vi "DataTranslation_Differential.vi"() -> ()   [LabVIEW 2011]
uses:
  Globals/Meas_global.vi
  PWA/PWAtasksGLOBAL.vi
  Data_Translation/DataTranslation_global.vi
  <userlib>/LV-Link3/PolySubVIs/DtOLTimingSetInput.vi
  <userlib>/LV-Link3/PolySubVIs/DtCreateAinChan.vi
  <userlib>/LV-Link3/PolySubVIs/DtOLReadMultiple2D.vi
  <userlib>/LV-Link3/PolySubVIs/DtOLTriggerDigital.vi
panel:
  out "Waveform Graph":dbl[][](graph)
  out "error out":errorcluster={"status"=TRUE, "code"=1172, "source"="Error calling method LvLink2.LvTask.ReadDblData2DAs1D, (System.Reflection.TargetInvocationException: Exception has been thrown by the target of an invocation.\n\tInner Exception: LvLink2.LvException: Timeout) <append><b>LvLink2.LvException</b> in OLReadMultiple2D.vi->DataTranslation_server.vi->Acquire_Data.vi->Get_data.vi->Measurement.vi"}
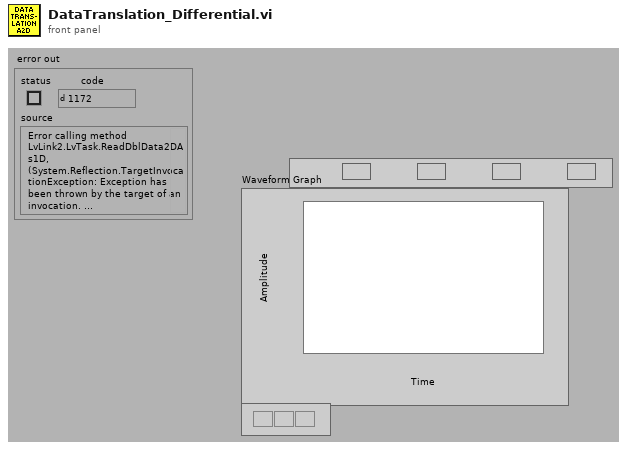
[diagram p1: front panel]
types:
  T1 = typedef "Ch_and_Spans.ctl" = cluster{"high limit (10V)":sgl, "low limit (-10V)":sgl, "Ch No":i16, "Var name":string, "Use Latest Calib":bool}
  T2 = typedef "Trigger_Mode.ctl" = enum16{"Free Running", "Start on Trigger", "Trigger Every Block", "Trigger Every Sample"}
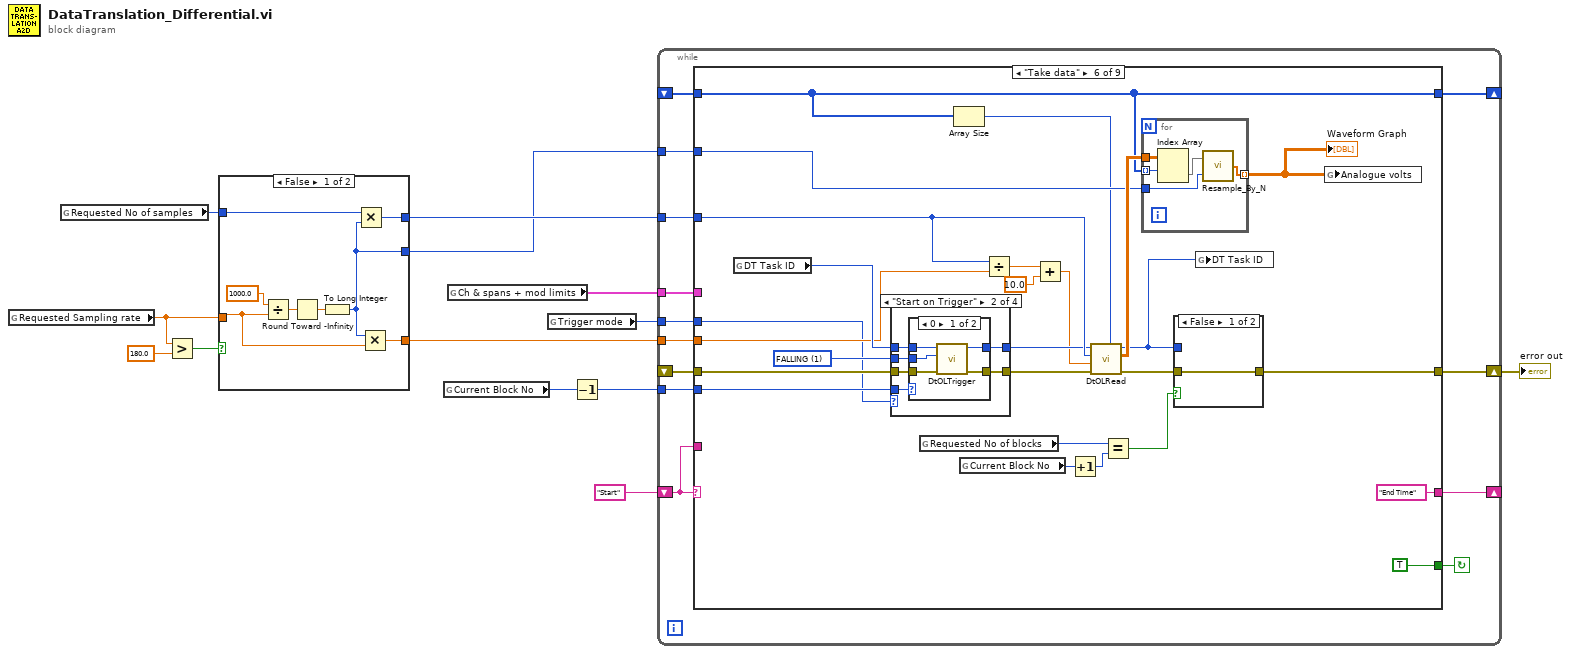
[diagram p0: block diagram]
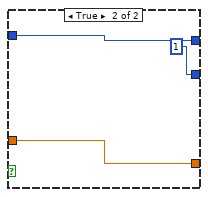
[diagram p2: hidden frame]
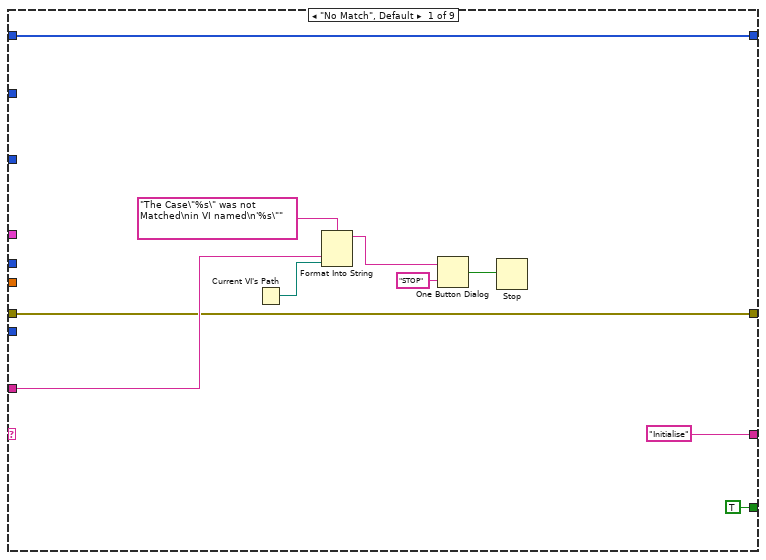
[diagram p3: hidden frame]
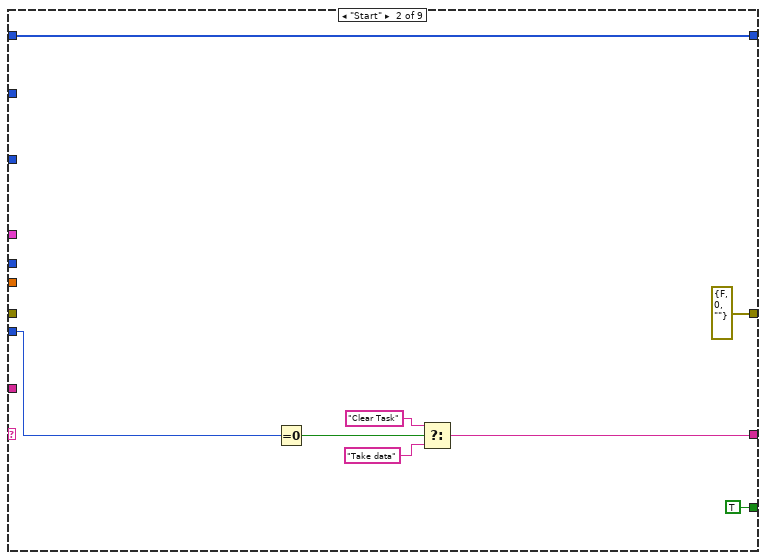
[diagram p4: hidden frame]
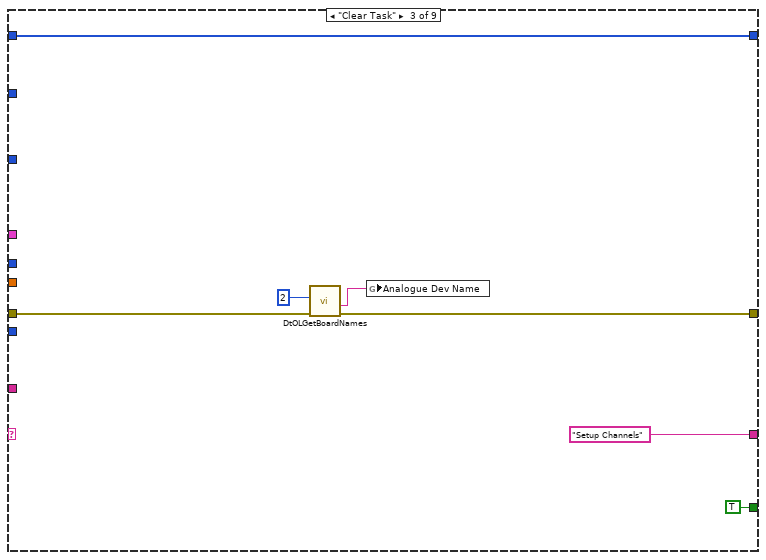
[diagram p5: hidden frame]
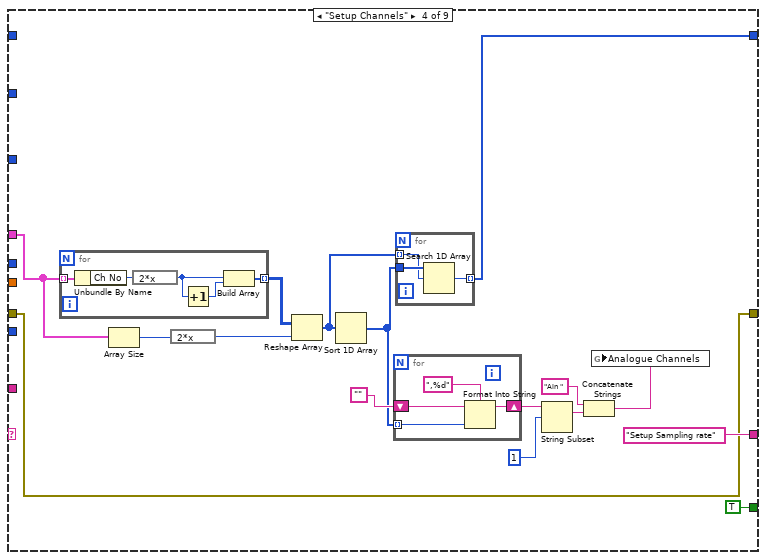
[diagram p6: hidden frame]
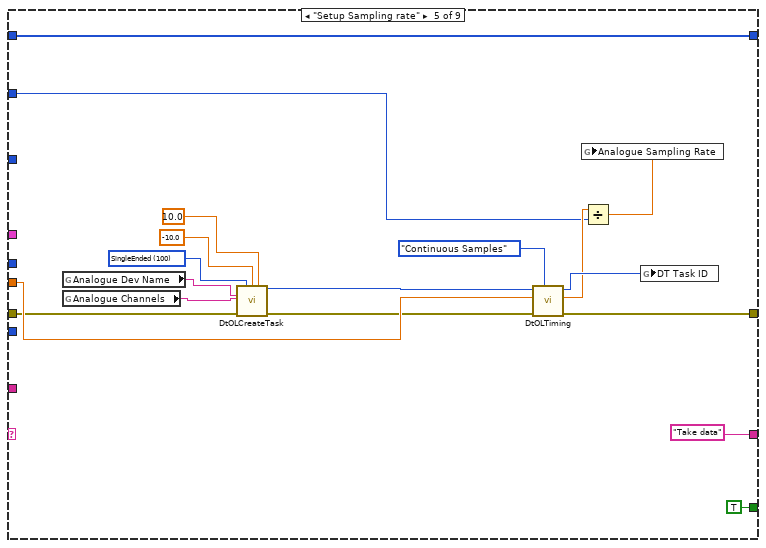
[diagram p7: hidden frame]
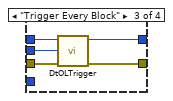
[diagram p10: hidden frame]
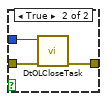
[diagram p12: hidden frame]
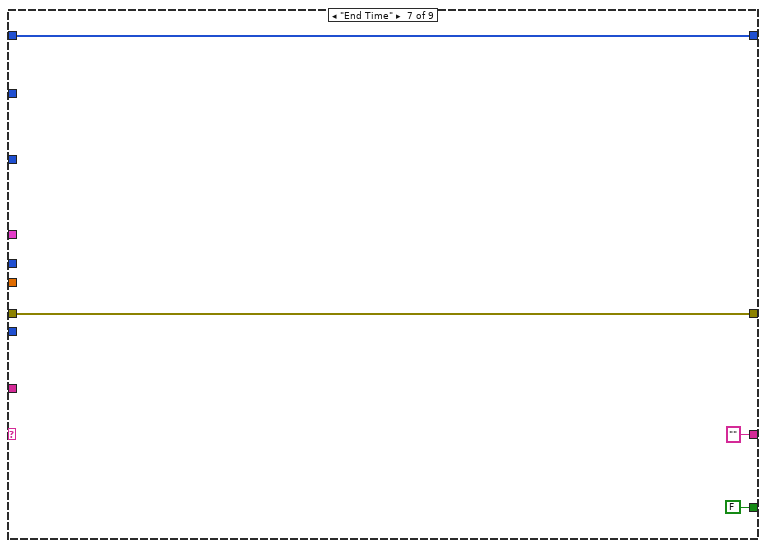
[diagram p13: hidden frame]
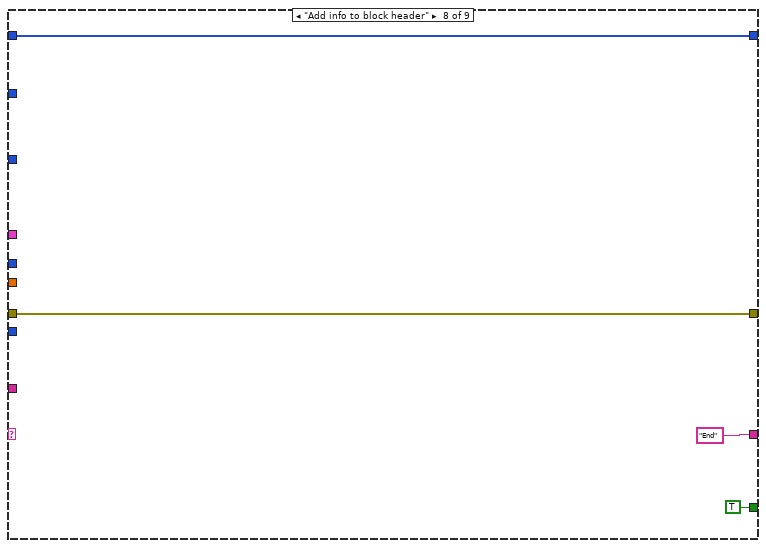
[diagram p14: hidden frame]
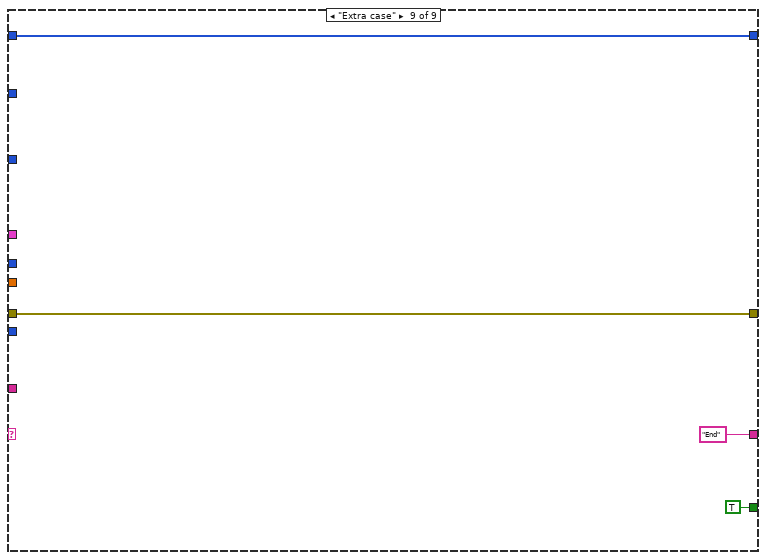
[diagram p15: hidden frame]
diagram:
  n1 = global read "Meas_global.vi" "Requested Sampling rate"() -> (w5:dbl)
  n2 = global read "Meas_global.vi" "Requested No of samples"() -> (w2:i32)
  n3 = Greater?(x=w5, y=180.0) -> (0:w10:bool)
  n4 = case shown="False" w10 {
    tunnel: w5 -> [w15 w24]
    tunnel: [w16 w24] -> w9
    tunnel: [w18 w23] -> w8
    tunnel: w2 -> [w17 w23]
    tunnel: [w14 1] -> w7
    frame False {
      n5 = Divide(x=1000.0, y=w15) -> (x/y=w20:dbl)
      n6 = Round Toward -Infinity(1:w20) -> (0:w19:dbl)
      n7 = To Long Integer(number=w19) -> (32bit integer=w14:i32)
      n8 = Multiply(x=w17, y=w14) -> (x*y=w18:i32)
      n9 = Multiply(x=w14, y=w15) -> (x*y=w16:dbl)
    }
    frame True {
    }
  }
  n10 = global read "Meas_global.vi" "Current Block No"() -> (w4:i32)
  n11 = global read "Meas_global.vi" "Ch & spans + mod limits"() -> (w6:T1[])
  n12 = global read "Meas_global.vi" "Trigger mode"() -> (w1:T2)
  n13 = Decrement(x=w4) -> (x-1=w3:i32)
  n14 = while {
    shift-left: "Start" -> [w36]
    shift-right: [w37] -> _
    shift-right: [w30] -> w12
    shift-left: _ -> [w35]
    tunnel: w9 -> [w34]
    tunnel: w8 -> [w33]
    tunnel: w3 -> [w32]
    tunnel: w6 -> [w31]
    shift-right: [w29] -> _
    shift-left: _ -> [w28]
    tunnel: w7 -> [w27]
    tunnel: w1 -> [w25]
    stop <- w26 continue-if-true
    n15 = case shown="\"Take data\"" w36 {
      tunnel: ["Initialise" w53 "Setup Channels" "Setup Sampling rate" "Take data" "End Time" "" ("f") "End" ("f") "End" ("f")] -> w37
      tunnel: w36 -> [w43 _ _ _ _ _ _ _ _]
      tunnel: [w40 errorcluster {"status"=FALSE, "code"=0, "source"=""} ("error out") w57 w72 w108 w119 w169 w172 w176] -> w30
      tunnel: w35 -> [w40 _ w58 w72 w94 w133 w169 w172 w176]
      tunnel: w34 -> [_ _ _ _ w107 w129 _ _ _]
      tunnel: w33 -> [_ _ _ _ _ w130 _ _ _]
      tunnel: w32 -> [_ w55 _ _ _ w128 _ _ _]
      tunnel: w31 -> [_ _ _ w66 _ _ _ _ _]
      tunnel: [w39 w51 w61 w74 w105 w127 w168 w171 w175] -> w29
      tunnel: w28 -> [w39 w51 w61 _ w105 w127 w168 w171 w175]
      tunnel: w27 -> [_ _ _ _ w102 w126 _ _ _]
      tunnel: [TRUE TRUE TRUE TRUE TRUE TRUE FALSE TRUE TRUE] -> w26
      tunnel: w25 -> [_ _ _ _ _ w111 _ _ _]
      frame "No Match", Default {
        (unwired) FALSE
        n16 = Current VI's Path() -> (path=w42:path)
        n17 = Format Into String(format string="The Case\"%s\" was not Matched\nin VI named\n'%s\"" ("Format String"), w43, w42) -> (resulting string=w46:string)  [unwired: 2 in, 1 out]
        n18 = One Button Dialog(message=w46, button name ("OK")="STOP") -> (true=w44:bool)
        n19 = Stop(stop? (T)=w44) -> ()
      }
      frame "Start" {
        (unwired) TRUE
        n20 = Equal To 0?(x=w55) -> (x = 0?=w54:bool)
        n21 = Select(t="Clear Task", s=w54, f="Take data") -> (s? t:f=w53:string)
      }
      frame "Clear Task" {
        (unwired) TRUE
        n22 = call <userlib>:"DtOLGetBoardNames.vi"("error in (no error)"=w58, "Select Board"=u32 2) -> ("error out"=w57:errorcluster, "Board Name"=w59:string)  [unwired: 7 in, 1 out]
        n23 = global write "PWAtasksGLOBAL.vi" "Analogue Dev Name"(w59) -> ()
      }
      frame "Setup Channels" {
        (unwired) TRUE
        n24 = for {
          tunnel: [w89] -> w69 mode=indexing
          tunnel: w66 -> [w88] mode=indexing
          n25 = Unbundle By Name(w88) -> ("Ch No"=w87:i16)
          n26 = expression code="2*x"(w87) -> (w86:i16)
          n27 = Increment(x=w86) -> (x+1=w90:i16)
          n28 = Build Array(w86, w90) -> (w89:i16[])
        }
        n29 = Array Size(array=w66) -> (size(s)=w68:i32)
        n30 = expression code="2*x"(w68) -> (w67:i32)
        n31 = Reshape Array(w69, w67) -> (w65:i16[])
        n32 = Sort 1D Array(array=w65) -> (sorted array=w63:i16[])
        n33 = for {
          shift-right: [w80] -> w64
          shift-left: "" -> [w81]
          tunnel: w63 -> [w79] mode=indexing
          n34 = Format Into String(format string=",%d", initial string=w81, w79) -> (resulting string=w80:string)  [unwired: 1 in, 1 out]
        }
        n35 = for {
          tunnel: w63 -> [w85]
          tunnel: w65 -> [w84] mode=indexing
          tunnel: [w83] -> w74 mode=indexing
          n36 = Search 1D Array(1D array=w85, element=w84) -> (index of element=w83:i32)  [unwired: 1 in]
        }
        n37 = String Subset(string=w64, offset (0)=1) -> (substring=w76:string)  [unwired: 1 in]
        n38 = Concatenate Strings("Ain ", w76) -> (w71:string)
        n39 = global write "Meas_global.vi" "Analogue Channels"(w71) -> ()
      }
      frame "Setup Sampling rate" {
        w96 = 100 items=["SingleEnded"=100, "Differential"=101] ("Channel Type")
        n40 = global read "PWAtasksGLOBAL.vi" "Analogue Dev Name"() -> (w95:string)
        n41 = global read "Meas_global.vi" "Analogue Channels"() -> (w91:string)
        n42 = call-poly <userlib>:"DtOLCreateTask.vi"("Channel Type"=w96, "Range Min"=-10.0, "Range Max"=10.0, "Board Name"=w95, "Channel"=w91, "error in (no error)"=w94) -> ("Task out"=w92:i32, "error out"=w93:errorcluster)  [unwired: 7 in, 1 out]
        n43 = call-poly <userlib>:"DtOLTiming.vi"("Sample Mode"=enum16{"Finite Samples", "Continuous Samples"}."Continuous Samples", "error in (no error)"=w93, "Sample Freq (Hz)"=w107, "Task in"=w92) -> ("error out"=w108:errorcluster, "Actual Sample Freq"=w103:dbl, "Task out"=w106:i32)  [unwired: 4 in, 1 out]
        n44 = Divide(x=w103, y=w102) -> (x/y=w101:dbl)
        n45 = global write "Meas_global.vi" "Analogue Sampling Rate"(w101) -> ()
        n46 = global write "DataTranslation_global.vi" "DT Task ID"(w106) -> ()
      }
      frame "Take data" {
        w112 = 1 items=["RISING", "FALLING"] ("External Trigger Polarity")
        n47 = global read "DataTranslation_global.vi" "DT Task ID"() -> (w132:i32)
        n48 = case shown="\"Start on Trigger\"" w111 {
          tunnel: [w136 w139 w153 w156] -> w116
          tunnel: w132 -> [w136 w141 w154 w156]
          tunnel: [w135 w138 w151 w155] -> w114
          tunnel: w133 -> [w135 w140 w152 w155]
          tunnel: w128 -> [_ w142 _ _]
          tunnel: w112 -> [_ w137 w150 _]
          frame "Free Running" {
          }
          frame "Start on Trigger" {
            n49 = case shown="0" w142 {
              tunnel: w141 -> [w147 w149]
              tunnel: w140 -> [w146 w148]
              tunnel: [w144 w149] -> w139
              tunnel: [w145 w148] -> w138
              tunnel: w137 -> [w143 _]
              frame 0 {
                n50 = call-poly <userlib>:"DtOLTrigger.vi"("error in (no error)"=w146, "External Trigger Polarity"=w143, "Task in"=w147) -> ("error out"=w145:errorcluster, "Task out"=w144:i32)  [unwired: 7 in]
              }
              frame 1, Default {
              }
            }
          }
          frame "Trigger Every Block" {
            n51 = call-poly <userlib>:"DtOLTrigger.vi"("error in (no error)"=w152, "External Trigger Polarity"=w150, "Task in"=w154) -> ("error out"=w151:errorcluster, "Task out"=w153:i32)  [unwired: 7 in]
          }
          frame "Trigger Every Sample" {
          }
        }
        n52 = global read "Meas_global.vi" "Requested No of blocks"() -> (w123:i32)
        n53 = Array Size(array=w127) -> (size(s)=w109:i32)
        n54 = global read "Meas_global.vi" "Current Block No"() -> (w125:i32)
        n55 = Divide(x=w130, y=w129) -> (x/y=w117:dbl)
        n56 = Add(x=w117, y=10.0) -> (x+y=w115:dbl)
        n57 = Increment(x=w125) -> (x+1=w124:i32)
        n58 = call-poly <userlib>:"DtOLRead.vi"("Number Chan to Read"=w109, "error in (no error)"=w114, "Timeout"=w115, "Samples Per Channel"=w130, "Task in"=w116) -> ("error out"=w120:errorcluster, "2D Data out"=w131:dbl[][], "Task out"=w122:i32)  [unwired: 2 in, 2 out]
        n59 = Equal?(x=w123, y=w124) -> (x = y?=w121:bool)
        n60 = for {
          tunnel: w127 -> [w165] mode=indexing
          tunnel: w131 -> [w164]
          tunnel: [w162] -> w110 mode=indexing
          tunnel: w126 -> [w161]
          n61 = Index Array(array=w164, index (row)=w165) -> (element=w163:dbl[])  [unwired: 1 in]
          n62 = call "Resample_By_N.vi"("Resample Factor"=w161, "Array In"=w163) -> ("Array Out"=w162:dbl[])
        }
        "Waveform Graph" <- w110
        n63 = case shown="False" w121 {
          tunnel: w122 -> [_ w160]
          tunnel: w120 -> [w157 w159]
          tunnel: [w157 w158] -> w119
          frame False {
          }
          frame True {
            n64 = call <userlib>:"DtOLCloseTask.vi"("Error in"=w159, "Task in"=w160) -> ("Error Out"=w158:errorcluster)  [unwired: 9 in]
          }
        }
        n65 = global write "DataTranslation_global.vi" "DT Task ID"(w122) -> ()
        n66 = global write "Meas_global.vi" "Analogue volts"(w110) -> ()
      }
      frame "End Time" {
      }
      frame "Add info to block header" {
      }
      frame "Extra case" {
        (unwired) FALSE
      }
    }
  }
  "error out" <- w12
